vi "Tacking Function.vi"() -> ()   [LabVIEW 2011]
uses:
  2 Typedefs/UTM Location.ctl
  2 Typedefs/Velocity.ctl
  <vilib>/Analysis/NI_AAL_Angle.lvlib
  <vilib>/Analysis/coordinate.llb/Absolute Angle Difference (scalar).vi
  0x2-OCU-Think Comm/0x2 Typedefs/ocuWaypoint.ctl
panel:
  out "reversed array":T1[](array[typedef]) {"UTM Location"."North" format="%#_10f"; "UTM Location"."East" format="%#_8f"}
  out "Good to Tack":bool
  out "Jump Length (m)":dbl
  in  "Wind Vector\nScaling Factor":dbl
  out "Tack Waypoint Plot":cluster{"Y":dbl[], "Y":dbl[]}[](graph)
  in  "Minimum Final\nTack Distance (m?)":dbl
  out "Number of jumps":dbl
  out "Angle from boat to waypoint (rad)":dbl
  in  "Bounding box\nside length (m?)":dbl
  out "Wind Direction (green)\nIrons (black)\nMax_angle (blue)\nMin_angle (red)":cluster{dbl, dbl, dbl, dbl}(knob) scale=-3.14..6.28
  # "QUIRK : If the 'Bounding box\nside length is 0 (as on opening)\nthe vi will go into an infinite loop"
  # "Also, you can't see the wind vector\nuntil this scaling factor is non-zero\n(10 - 30 is good)"
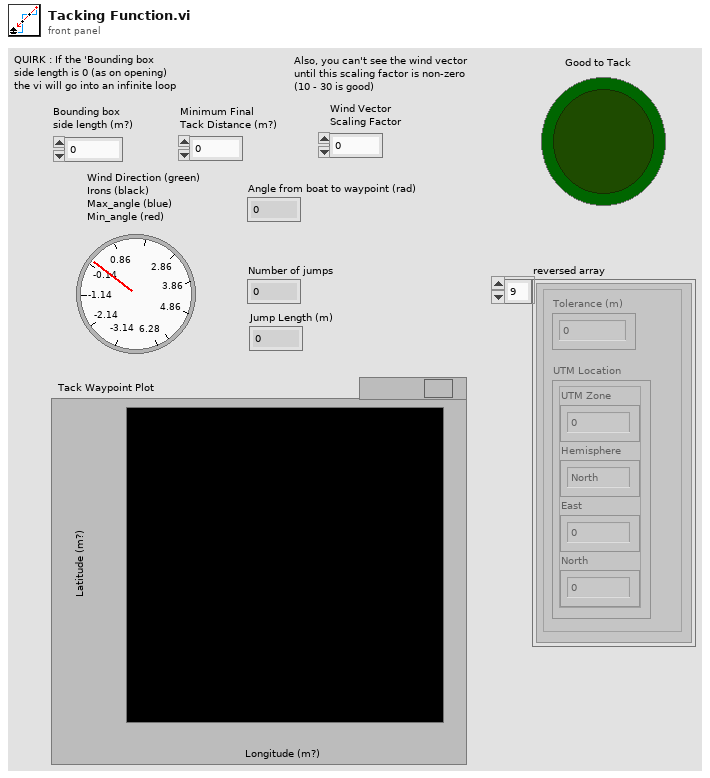
[diagram p1: front panel]
types:
  T1 = typedef "ocuWaypoint.ctl" = cluster{"Tolerance (m)":dbl, "UTM Location":T2}
  T2 = typedef "UTM Location.ctl" = cluster{"UTM Zone":dbl, "Hemisphere":enum16{"North", "South"}, "East":dbl, "North":dbl}
  T3 = typedef "Velocity.ctl" = cluster{"East":dbl, "North":dbl}
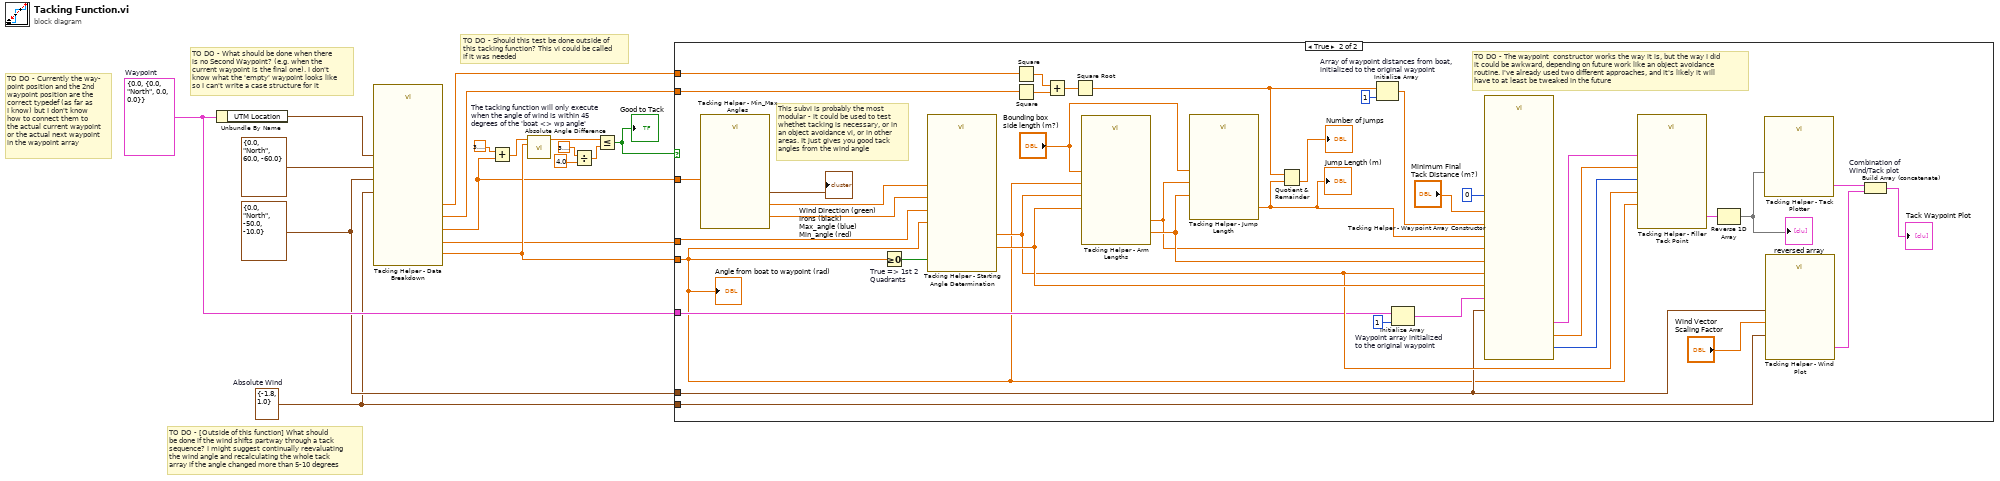
[diagram p0: block diagram]
diagram:
  w1 = T3 {"East"=-1.8, "North"=1.0}  # Absolute Wind
  w3 = T2 {"UTM Zone"=0.0, "Hemisphere"=enum."North", "East"=-50.0, "North"=-10.0} ("Robot UTM Location")
  w4 = T1 {"Tolerance (m)"=0.0, "UTM Location"={"UTM Zone"=0.0, "Hemisphere"=enum."North", "East"=0.0, "North"=0.0}}  # Waypoint
  # "TO DO - Should this test be done outside of\nthis tacking function? This vi could be called\nif it was needed"
  # "TO DO - Currently the way-\npoint position and the 2nd\nwaypoint position are the\ncorrect typedef (as far as\nI know) but I don't know\nhow to connect them to\nthe actual current waypoint\nor the actual next waypoint\nin the waypoint array"
  # "TO DO - [Outside of this function] What should\nbe done if the wind shifts partway through a tack\nsequence? I might suggest continually reevaluating\nthe wind angle and recalculating the whole tack\narray if the angle changed more than 5-10 degrees"
  # "TO DO - What should be done when there\nis no Second Waypoint? (e.g. when the\ncurrent waypoint is the final one). I don't\nknow what the 'empty' waypoint looks like\nso I can't write a case structure for it"
  n1 = Unbundle By Name(w4) -> ("UTM Location"=w8:T2)
  n2 = call "Tacking Helper - Data Breakdown.vi"("Absolute\nWind Vector"=w1, "Second\nWaypoint\nPosition"=T2 {"UTM Zone"=0.0, "Hemisphere"=enum."North", "East"=60.0, "North"=-60.0} ("UTM Location"), "Boat\nPosition"=w3, "Waypoint\nPosition"=w8) -> ("Angle of Wind"=w10:dbl, "X, boat > wp"=w6:dbl, "Y, boat >wp"=w5:dbl, "Boat <> 2nd wp Angle"=w7:dbl, "Boat <> wp Angle"=w17:dbl)  [unwired: 3 in]
  n3 = Add(x=3.141592653589793, y=w10) -> (x+y=w16:dbl)
  n4 = call-poly <vilib>:"Absolute Angle Difference.vi"("angle 2"=w17, "angle 1"=w16) -> ("absolute angle difference"=w15:dbl)  [unwired: 8 in, 1 out]
  n5 = Divide(x=3.141592653589793, y=4.0) -> (x/y=w12:dbl)
  n6 = Less Or Equal? "The tacking function will only execute\nwhen the angle of wind is within 45\ndegrees of the 'boat <> wp angle'"(x=w15, y=w12) -> (x <= y?=w11:bool)
  "Good to Tack" <- w11
  n7 = case shown="True" w11 {
    tunnel: w7 -> [_ w28]
    tunnel: w6 -> [_ w54]
    tunnel: w5 -> [_ w53]
    tunnel: w4 -> [_ w21]
    tunnel: w10 -> [_ w47]
    tunnel: w17 -> [_ w20]
    tunnel: w3 -> [_ w22]
    tunnel: w1 -> [_ w39]
    frame False {
    }
    frame True {
      # "TO DO - The waypoint  constructor works the way it is, but the way I did\nit could be awkward, depending on future work like an object avoidance\nroutine. I've already used two different approaches, and it's likely it will\nhave to at least be tweaked in the future"
      # "This subvi is probably the most\nmodular - it could be used to test\nwhethet tacking is necessary, or in\nan object avoidance vi, or in other\nareas. It just gives you good tack\nangles from the wind angle"
      n8 = call "Tacking Helper - Min_Max Angles.vi"("Wind Direction (rad)"=w47) -> ("Irons/Tack\nIndicator"=→"Wind Direction (green)\nIrons (black)\nMax_angle (blue)\nMin_angle (red)":cluster{dbl, dbl, dbl, dbl}, "Max Angle\nof Tack"=w35:dbl, "Min Angle\nof Tack"=w34:dbl)  [unwired: 8 in]
      n9 = Greater Or Equal To 0? "True => 1st 2\nQuadrants"(x=w20) -> (x >= 0?=w46:bool)
      n10 = call "Tacking Helper - Starting Angle Determination.vi"("Boat <> 2nd wp Angle"=w28, "Is the boat to wp\nangle greater than 0?"=w46, "Max Angle\nof Tack"=w35, "Min Angle\nof Tack"=w34, "Angle from boat to waypoint"=w20) -> ("Second Angle"=w24:dbl, "Starting Angle"=w23:dbl)  [unwired: 5 in]
      n11 = Square(x=w54) -> (x^2=w52:dbl)
      n12 = Square(x=w53) -> (x^2=w51:dbl)
      n13 = Add(x=w52, y=w51) -> (x+y=w50:dbl)
      n14 = Square Root(x=w50) -> (sqrt(x)=w38:dbl)
      n15 = call "Tacking Helper - Arm Lengths.vi"("Bounding box\nside length (m?)"="Bounding box\nside length (m?)", "Second Angle"=w24, "Starting Angle"=w23, "Angle from boat\nto waypoint"=w20) -> ("Second\nArm Length"=w45:dbl, "Starting\nArm Length"=w31:dbl)  [unwired: 6 in]
      n16 = call "Tacking Helper - Jump Length.vi"("Bounding box\nside length (m?)"="Bounding box\nside length (m?)", "Second\nArm Length"=w45, "Starting\nArm Length"=w31) -> ("Jump Length (m)"=w32:dbl)  [unwired: 8 in]
      "Jump Length (m)" <- w32
      n17 = Quotient & Remainder(x=w38, y=w32) -> (floor(x/y)=→"Number of jumps":dbl)  [unwired: 1 out]
      n18 = Initialize Array "Array of waypoint distances from boat,\ninitialized to the original waypoint"(w38, 1 ("dimension size")) -> (w42:dbl[])
      n19 = Initialize Array "Waypoint array initialized\nto the original waypoint"(w21, 1 ("dimension size")) -> (w44:T1[])
      n20 = call "Tacking Helper - Waypoint Array Constructor.vi"("Second Angle"=w24, "Minimum Final Tack Distance (m?)"="Minimum Final\nTack Distance (m?)", "Starting\nArm Length"=w31, "Second\nArm Length"=w45, "Jump Length (m)"=w32, "Starting Angle"=w23, "Distance of each waypoint to boat"=w42, "Array Beginning"=0, "Waypoint Array In"=w44, "Boat Position"=w22) -> ("Distance to boat"=w26:dbl, "Final Index of\nWaypoint Array"=w27:i32, "Intermediate \nWaypoint Array out"=w25:T1[])  [unwired: 3 in]
      n21 = call "Tacking Helper - Filler Tack Point.vi"("Waypoint Array"=w25, "Distance to boat"=w26, "Final Index of Waypoint Array"=w27, "Starting Angle"=w23, "Angle from boat to waypoint"=w20) -> ("Finalized Waypoint Array"=w19:T1[])  [unwired: 6 in]
      n22 = Reverse 1D Array(array=w19) -> (reversed array=w18:T1[])
      "reversed array" <- w18
      n23 = call "Tacking Helper - Tack Plotter.vi"("Intermediate\nWaypoints In"=w18) -> ("Tack Plot Data Out"=w41:cluster{dbl[], dbl[]}[])  [unwired: 10 in]
      n24 = call "Tacking Helper - Wind Plot.vi"("Boat\nPosition"=w22, "Wind Vector\nTop = x\nBottom = y"=w39, "Wind Vector\nScaling Factor"="Wind Vector\nScaling Factor") -> ("Output Cluster\nFor Plotting"=w36:cluster{dbl[], dbl[]})  [unwired: 8 in]
      n25 = Build Array (concatenate) "Combination of\nWind/Tack plot"(w41, w36) -> (→"Tack Waypoint Plot":cluster{dbl[], dbl[]}[])
      "Angle from boat to waypoint (rad)" <- w20
    }
  }
